vi "FlatSequence.vi"() -> ()   [LabVIEW 2019]
panel:
  out "Numeric 2":i32
  out "Numeric":i32
  in  "stop 2":bool
  in  "stop":bool
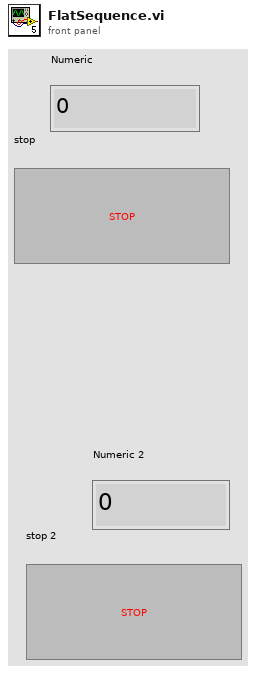
[diagram p1: front panel]
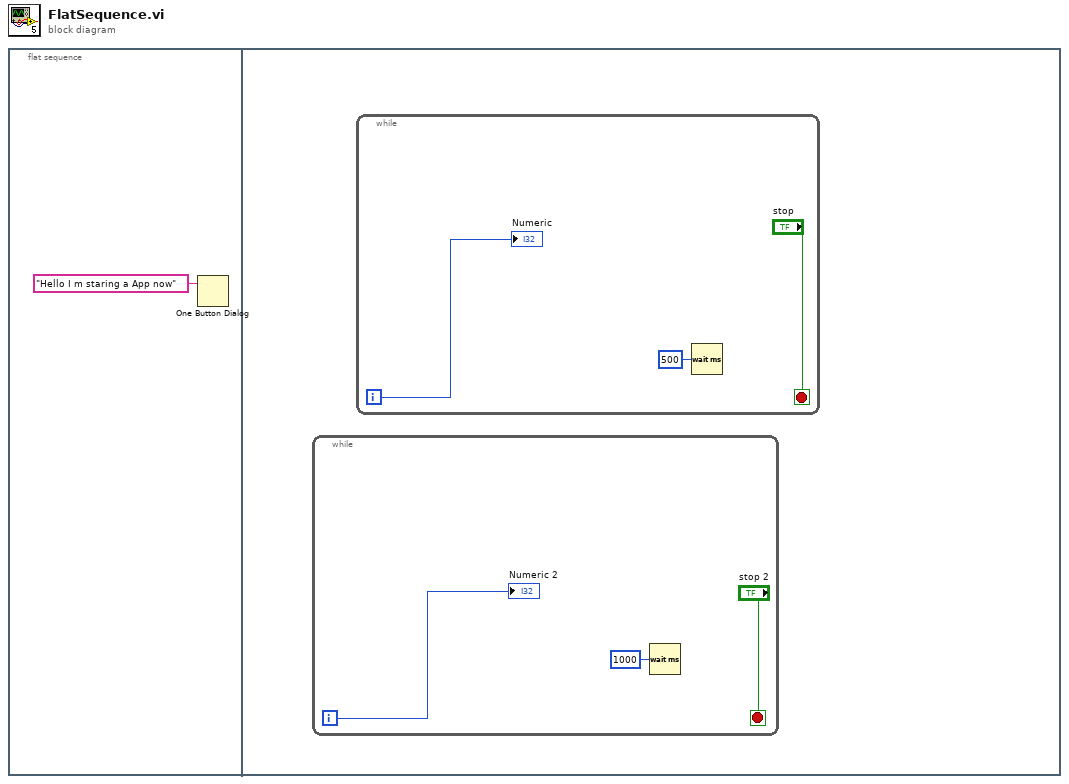
[diagram p0: block diagram]
diagram:
  n1 = flat-sequence {
    frame #0 {
      n2 = One Button Dialog(message="Hello I m staring a App now") -> ()  [unwired: 1 in, 1 out]
    }
    frame #1 {
      n3 = while {
        i -> [w3]
        stop <- "stop 2" stop-if-true
        n4 = Wait (ms)(milliseconds to wait=u32 1000) -> ()  [unwired: 1 out]
        "Numeric 2" <- w3
      }
      n5 = while {
        i -> [w6]
        stop <- "stop" stop-if-true
        n6 = Wait (ms)(milliseconds to wait=u32 500) -> ()  [unwired: 1 out]
        "Numeric" <- w6
      }
    }
  }
